vi "Channels FGV.vi"(9 "SSD1306 Channels":T1, 11 "SSD1306 FGV State":T2) -> (1 "SSD1306 Channels":T1)   [LabVIEW 2020, in "LMH-LINX.lvlib" / "SSD1306.lvlib"]
uses:
  SSD1306.lvlib
  SSD1306 FGV State.ctl
  SSD1306 Config.ctl
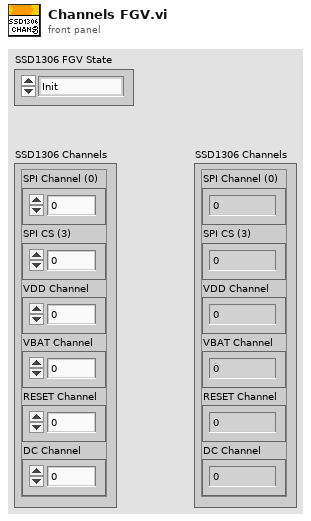
[diagram p1: front panel]
types:
  T1 = typedef "LMH-LINX.lvlib/SSD1306.lvlib/SSD1306 Config.ctl" = cluster{"SPI Channel (0)":u8, "VDD Channel":u8, "VBAT Channel":u8, "RESET Channel":u8, "DC Channel":u8, "SPI CS (3)":u8}
  T2 = typedef "LMH-LINX.lvlib/SSD1306.lvlib/SSD1306 FGV State.ctl" = enum16{"Init", "Set", "Get"}
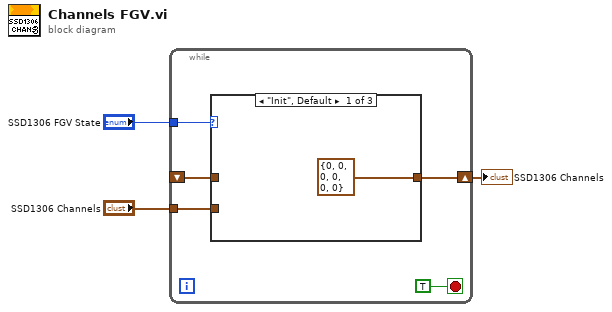
[diagram p0: block diagram]
diagram:
  n1 = while {
    tunnel: "SSD1306 FGV State" -> [w8]
    shift-right: [w7] -> w1
    shift-left: _ -> [w6]
    tunnel: "SSD1306 Channels" -> [w4]
    stop <- TRUE stop-if-true
    n2 = case shown="\"Init\", Default" w8 {
      tunnel: [T1 {"SPI Channel (0)"=0, "VDD Channel"=0, "VBAT Channel"=0, "RESET Channel"=0, "DC Channel"=0, "SPI CS (3)"=0} ("SSD1306 Channels") w10 w11] -> w7
      tunnel: w6 -> [_ _ w11]
      tunnel: w4 -> [_ w10 _]
      frame "Init", Default {
      }
      frame "Set" {
      }
      frame "Get" {
      }
    }
  }
  "SSD1306 Channels" <- w1
